vi "WebSocket Server.vi"(8 "error in (no error)":errorcluster, 9 "Handler References":variant, 10 "Configuration":T1={"Listen Port"=7890, "Handler Ref"=refnum}, 11 "Main Event":refnum<user-event>) -> (0 "error out":errorcluster)   [LabVIEW 2013, in "WebSocket Server.lvlib"]
uses:
  WebSocket Server.lvlib
  <vilib>/Intelligent Energy/Message Queue Helper/ctl_QMH_Message_Typedef.ctl
  ctl_Configuration.ctl
  <vilib>/Intelligent Energy/Message Queue Helper/MessageQueueHelper.lvlib
panel:
  out "Listen Port":u16
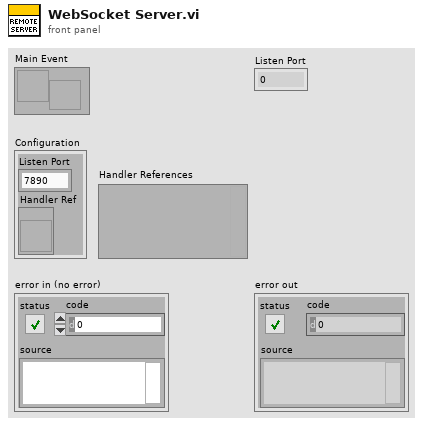
[diagram p1: front panel]
types:
  T1 = typedef "WebSocket Server.lvlib/ctl_Configuration.ctl" = cluster{"Listen Port":u16, "Handler Ref":refnum<vi>}
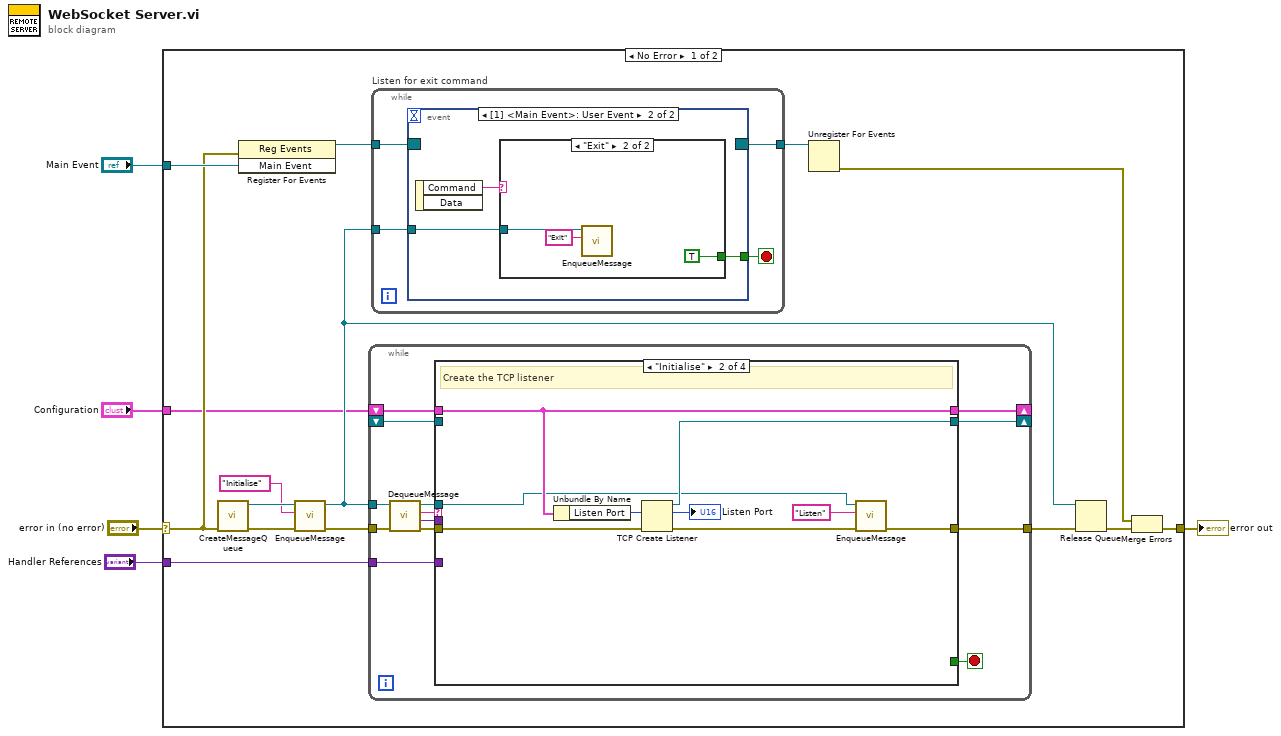
[diagram p0: block diagram]
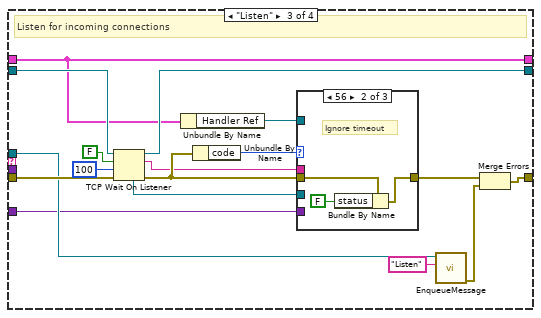
[diagram p3: hidden frame]
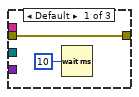
[diagram p4: hidden frame]
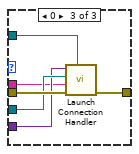
[diagram p5: hidden frame]
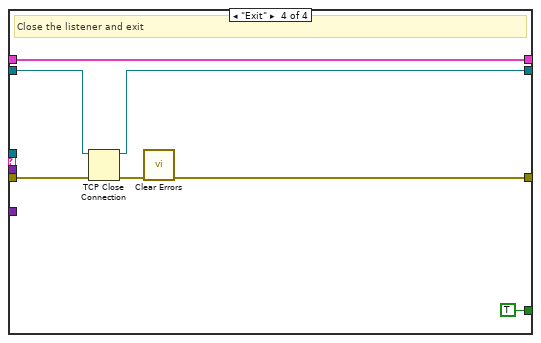
[diagram p6: hidden frame]
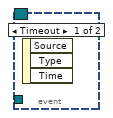
[diagram p7: hidden frame]
diagram:
  n1 = case shown="No Error" "error in (no error)" {
    selector: "error in (no error)" -> [w8 w91]
    tunnel: [w11 w91] -> w5
    tunnel: "Main Event" -> [w9 _]
    tunnel: "Configuration" -> [w7 _]
    tunnel: "Handler References" -> [w6 _]
    frame No Error {
      n2 = call <vilib>:"CreateMessageQueue.vi"("error in (no error)"=w8) -> ("error out"=w18:errorcluster, "queue out"=w16:refnum<queue>)  [unwired: 8 in, 1 out]
      n3 = register-events(error in=w8, w9) -> (reference out=w20:refnum<event-registration>)  [unwired: 1 in, 1 out]
      n4 = call <vilib>:"EnqueueMessage.vi"("error in (no error)"=w18, "Message"="Initialise", "queue in"=w16) -> ("error out"=w17:errorcluster, "queue out"=w15:refnum<queue>)  [unwired: 7 in]
      n5 = while {
        tunnel: w15 -> [w33]
        tunnel: w17 -> [w32]
        tunnel: [w21] -> w14
        shift-right: [w25] -> _
        shift-left: w7 -> [w26]
        shift-right: [w24] -> _
        shift-left: _ -> [w23]
        tunnel: w6 -> [w22]
        stop <- w27 stop-if-true
        n6 = call <vilib>:"DequeueMessage.vi"("error in (no error)"=w32, "queue in"=w33) -> ("error out"=w30:errorcluster, "Data"=w28:variant, "Command"=w31:string, "queue out"=w29:refnum<queue>)  [unwired: 6 in]
        n7 = case shown="\"Initialise\"" w31 {
          tunnel: w30 -> [w36 w45 w62 w78]
          tunnel: [w36 w40 w51 w74] -> w21
          tunnel: w29 -> [_ w39 w56 _]
          tunnel: w28 -> [_ _ _ _]
          tunnel: [_ _ _ TRUE] -> w27
          tunnel: w26 -> [w35 w44 w48 w79]
          tunnel: [w35 w44 w48 w79] -> w25
          tunnel: [w34 w42 w59 w76] -> w24
          tunnel: w23 -> [w34 _ w61 w77]
          tunnel: w22 -> [_ _ w50 _]
          frame Default {
          }
          frame "Initialise" {
            # "Create the TCP listener"
            n8 = Unbundle By Name(w44) -> ("Listen Port"=w43:u16)
            n9 = TCP Create Listener(8:w45, 10:w43) -> (0:w41:errorcluster, 2:→"Listen Port":u16, 3:w42:refnum<k5>)  [unwired: 3 in]
            n10 = call <vilib>:"EnqueueMessage.vi"("error in (no error)"=w41, "Message"="Listen", "queue in"=w39) -> ("error out"=w40:errorcluster)  [unwired: 7 in, 1 out]
          }
          frame "Listen" {
            # "Listen for incoming connections"
            n11 = TCP Wait On Listener(8:w62, 9:100 ("timeout ms (wait forever: -1)"), 10:FALSE ("resolve remote address (T)"), 11:w61) -> (0:w57:errorcluster, 2:w49:string, 3:w59:refnum<k5>, 4:w54:refnum<k5>)  [unwired: 1 out]
            n12 = Unbundle By Name(w48) -> ("Handler Ref"=w47:refnum<vi>)
            n13 = Unbundle By Name(w57) -> ("code"=w58:i32)
            n14 = case shown="56" w58 {
              tunnel: w57 -> [w64 w67 w73]
              tunnel: [w64 w65 w72] -> w53
              tunnel: w54 -> [_ _ w71]
              tunnel: w50 -> [_ _ w70]
              tunnel: w49 -> [_ _ w69]
              tunnel: w47 -> [_ _ w68]
              frame Default {
                n15 = Wait (ms)(milliseconds to wait=u32 10) -> ()  [unwired: 1 out]
              }
              frame 56 {
                # "Ignore timeout"
                n16 = Bundle By Name(cluster=w67, "status"=FALSE) -> (w65:errorcluster)
              }
              frame 0 {
                n17 = call "Launch Connection Handler.vi"("Connection Handler Reference"=w68, "error in (no error)"=w73, "Remote Address"=w69, "WebSocket Connection in"=w71, "References In"=w70) -> ("error out"=w72:errorcluster)  [unwired: 6 in]
              }
            }
            n18 = call <vilib>:"EnqueueMessage.vi"("Message"="Listen", "queue in"=w56) -> ("error out"=w52:errorcluster)  [unwired: 8 in, 1 out]
            n19 = Merge Errors(w53, w52) -> (w51:errorcluster)
          }
          frame "Exit" {
            # "Close the listener and exit"
            n20 = TCP Close Connection(connection ID=w77, error in (no error)=w78) -> (connection ID out=w76:refnum<k5>, error out=w75:errorcluster)  [unwired: 1 in]
            n21 = call <vilib>:"Clear Errors.vi"("error in (no error)"=w75) -> ("error out"=w74:errorcluster)  [unwired: 6 in]
          }
        }
      }
      n22 = while "Listen for exit command" {
        tunnel: w20 -> [w84]
        tunnel: [w83] -> w19
        tunnel: w15 -> [w81]
        stop <- w82 stop-if-true
        n23 = event shown="[1] <Main Event>: User Event" {
          selector: w84 -> [_ _]
          dyn-events: [_ _] -> w83
          timeout: _ -> [_ _]
          tunnel: [_ w86] -> w82
          tunnel: w81 -> [_ w85]
          event Timeout {
            n24 = event-data() -> ()  [unwired: 1 in, 3 out]
          }
          event User Event {
            n25 = event-data() -> ("Command"=w87:string)  [unwired: 1 in, 1 out]
            n26 = case shown="\"Exit\"" w87 {
              tunnel: [_ TRUE] -> w86
              tunnel: w85 -> [_ w89]
              frame Default {
              }
              frame "Exit" {
                n27 = call <vilib>:"EnqueueMessage.vi"("Message"="Exit", "queue in"=w89) -> ()  [unwired: 8 in, 2 out]
              }
            }
          }
        }
      }
      n28 = Unregister For Events(event registration refnum=w19) -> (error out=w12:errorcluster)  [unwired: 1 in]
      n29 = Release Queue(queue=w15, error in (no error)=w14) -> (error out=w13:errorcluster)  [unwired: 1 in, 2 out]
      n30 = Merge Errors(w12, w13) -> (w11:errorcluster)
    }
    frame Error {
    }
  }
  "error out" <- w5
